vi "TestInfrared.vi"() -> ()   [LabVIEW 2016]
panel:
  out "IF readings (meters)":dbl[](array[numeric]) format="%_6g"
  in  "stop":bool
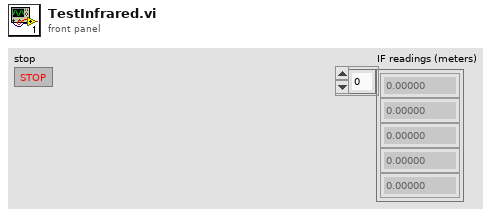
[diagram p1: front panel]
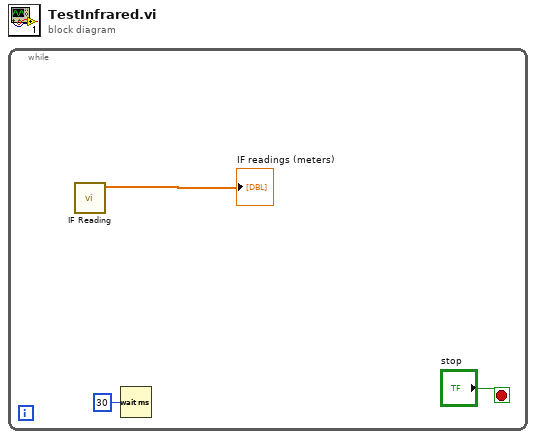
[diagram p0: block diagram]
diagram:
  n1 = while {
    stop <- "stop" stop-if-true
    n2 = call "IF Reading.vi"() -> ("IF readings (meters)"=→"IF readings (meters)":dbl[])  [unwired: 10 in, 1 out]
    n3 = Wait (ms)(milliseconds to wait=u32 30) -> ()  [unwired: 1 out]
  }
